vi "Creat Tags.vi"(1 "File Path":path=path "\\\\10file01\\RedirectedFolders/mike.delaplain/Documents/LabVIEW/SDF Small Gasifier/Tags_Dev.csv") -> (0 "CVT Tags":T1)   [LabVIEW 2013]
uses:
  <vilib>/NI/Current Value Table/Type Defs/Single Tag.ctl
  <vilib>/NI/Current Value Table/Type Defs/Data Types.ctl
  <vilib>/NI/Current Value Table/Type Defs/File Format.ctl
  <vilib>/NI/Current Value Table/Type Defs/Tag Grouping set.ctl
  <vilib>/Utility/file.llb/Read From Spreadsheet File (string).vi
  <vilib>/NI/Current Value Table/Current Value Table.lvlib
panel:
  out "CVT Tags":T2[](array[typedef])
  out "Invalid  CVT Tags":T2[](array[typedef])
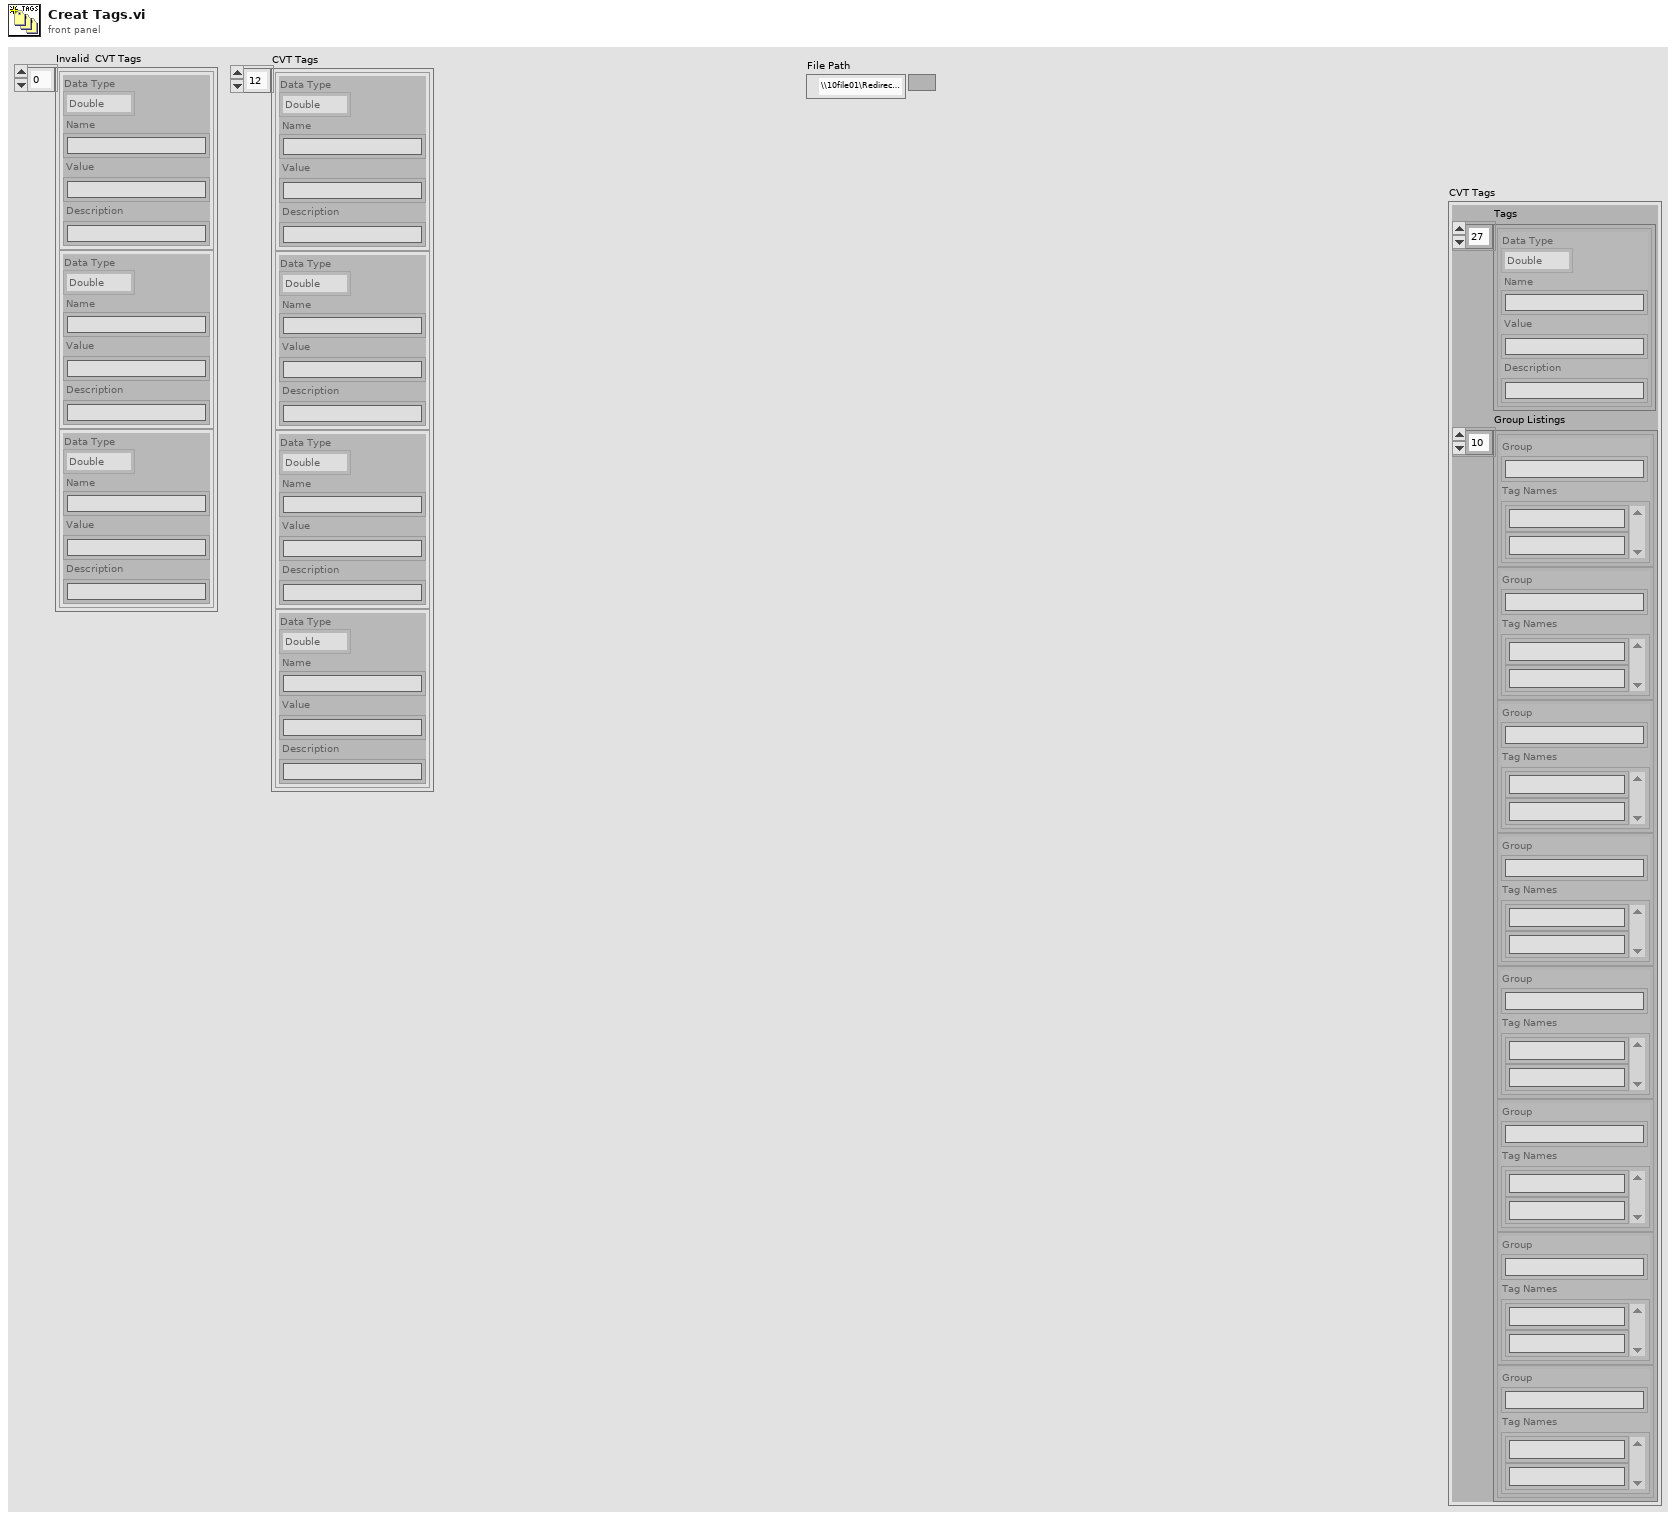
[diagram p1: front panel]
types:
  T1 = typedef "Current Value Table.lvlib/File Format.ctl" = cluster{"Tags":T2[], "Group Listings":T4[]}
  T2 = typedef "Current Value Table.lvlib/Single Tag.ctl" = cluster{"Data Type":T3, "Name":string, "Value":string, "Description":string}
  T3 = typedef "Current Value Table.lvlib/Data Types.ctl" = enum16{"Double", "Single", "I64", "I32", "I16", "I8", "U64", "U32", "U16", "U8", "String", "Boolean", "Array of U8", "Array of U16", "Array of U32", "Array of U64", "Array of I64", "Array of I32", "Array of I16", "Array of I8", "Array of Double", "Array of Single", "Array of Boolean", "Array of String"}
  T4 = typedef "Current Value Table.lvlib/Tag Grouping set.ctl" = cluster{"Group":string, "Tag Names":string[]}
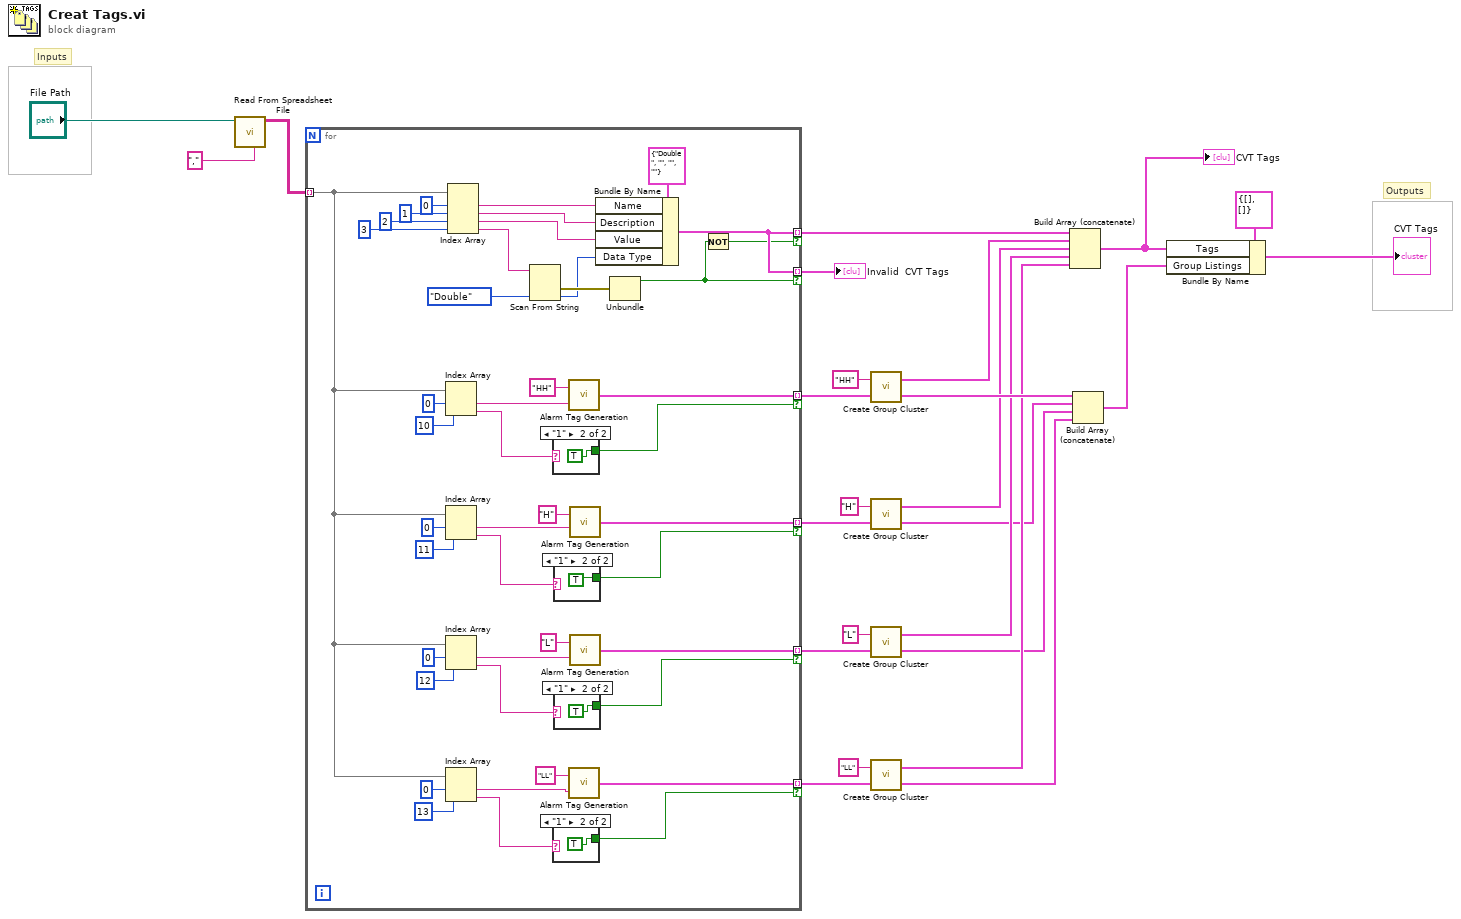
[diagram p0: block diagram]
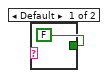
[diagram p2: hidden frame]
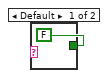
[diagram p3: hidden frame]
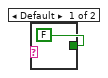
[diagram p4: hidden frame]
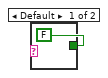
[diagram p5: hidden frame]
diagram:
  # "Inputs"
  # "Outputs"
  n1 = call-poly <vilib>:"Read From Spreadsheet File.vi"("delimiter (\\t)"="," ("delimiter (\\t)"), "file path (dialog if empty)"="File Path") -> ("all rows"=w20:string[][])  [unwired: 5 in, 4 out]
  n2 = for {
    tunnel: w20 -> [w44] mode=indexing
    tunnel: [w66] -> w22 mode=indexing if=w65
    tunnel: [w66] -> w18 mode=indexing if=w49
    tunnel: [w41] -> w15 mode=indexing if=w45
    tunnel: [w36] -> w9 mode=indexing if=w28
    tunnel: [w31] -> w8 mode=indexing if=w27
    tunnel: [w30] -> w7 mode=indexing if=w26
    n3 = Index Array(array=w44, index #1=0 ("index"), index #2=10 ("index")) -> (element #1=w42:string, element #2=w46:string)
    n4 = Index Array(array=w44, index #1=0 ("index"), index #2=11 ("index")) -> (element #1=w37:string, element #2=w29:string)
    n5 = Index Array(array=w44, index #1=0 ("index"), index #2=12 ("index")) -> (element #1=w35:string, element #2=w34:string)
    n6 = Index Array(array=w44, index #1=0 ("index"), index #2=13 ("index")) -> (element #1=w33:string, element #2=w32:string)
    n7 = Index Array(array=w44, index #1=0 ("index"), index #2=1 ("index"), index #3=2 ("index"), index #4=3 ("index")) -> (element #1=w68:string, element #2=w59:string, element #3=w58:string, element #4=w56:string)
    n8 = Scan From String(input string=w56, default 1=Data_Types."Double" ("Data Type")) -> (error out=w67:errorcluster, output 1=w57:T3)  [unwired: 3 in, 2 out]
    n9 = case shown="\"1\"" w46 {
      tunnel: [FALSE TRUE] -> w45
      frame Default {
      }
      frame "1" {
      }
    }
    n10 = case shown="\"1\"" w32 {
      tunnel: [FALSE TRUE] -> w26
      frame Default {
      }
      frame "1" {
      }
    }
    n11 = case shown="\"1\"" w29 {
      tunnel: [FALSE TRUE] -> w28
      frame Default {
      }
      frame "1" {
      }
    }
    n12 = case shown="\"1\"" w34 {
      tunnel: [FALSE TRUE] -> w27
      frame Default {
      }
      frame "1" {
      }
    }
    n13 = call "Alarm Tag Generation.vi"("Spreadsheet Input"=w42, "Alarm Type"="HH") -> ("Group & CVT Tag List"=w41:cluster{string[], T2[]})
    n14 = call "Alarm Tag Generation.vi"("Spreadsheet Input"=w33, "Alarm Type"="LL") -> ("Group & CVT Tag List"=w30:cluster{string[], T2[]})
    n15 = call "Alarm Tag Generation.vi"("Spreadsheet Input"=w37, "Alarm Type"="H") -> ("Group & CVT Tag List"=w36:cluster{string[], T2[]})
    n16 = call "Alarm Tag Generation.vi"("Spreadsheet Input"=w35, "Alarm Type"="L") -> ("Group & CVT Tag List"=w31:cluster{string[], T2[]})
    n17 = Bundle By Name(cluster=T2 {"Data Type"=enum."Double", "Name"="", "Value"="", "Description"=""} ("Tag"), "Name"=w68, "Description"=w59, "Value"=w58, "Data Type"=w57) -> (w66:T2)
    n18 = Unbundle(w67) -> ("status"=w65:bool)  [unwired: 2 out]
    n19 = Not(x=w65) -> (.not. x?=w49:bool)
  }
  "Invalid  CVT Tags" <- w22
  n20 = call "Create Group Cluster.vi"("Groups & Tags"=w15, "Alarm Type"="HH") -> ("CVT Groups"=w13:T4[], "CVT Tags"=w14:T2[])
  n21 = call "Create Group Cluster.vi"("Groups & Tags"=w9, "Alarm Type"="H") -> ("CVT Groups"=w3:T4[], "CVT Tags"=w6:T2[])
  n22 = call "Create Group Cluster.vi"("Groups & Tags"=w8, "Alarm Type"="L") -> ("CVT Groups"=w2:T4[], "CVT Tags"=w5:T2[])
  n23 = call "Create Group Cluster.vi"("Groups & Tags"=w7, "Alarm Type"="LL") -> ("CVT Groups"=w1:T4[], "CVT Tags"=w4:T2[])
  n24 = Build Array (concatenate)(w18, w14, w6, w5, w4) -> (w19:T2[])
  "CVT Tags" <- w19
  n25 = Build Array (concatenate)(w13, w3, w2, w1) -> (w17:T4[])
  n26 = Bundle By Name(cluster=T1 {"Tags"=[], "Group Listings"=[]} ("CVT Tags to Create"), "Tags"=w19, "Group Listings"=w17) -> (→"CVT Tags":T1)
